vi "Get About Information.vi"(8 "error in (no error)":errorcluster) -> (0 "error out":errorcluster, 3 "About vCE text Out":string)   [LabVIEW 2013, in "FPGADMAChannelData.lvclass"]
uses:
  FPGADMAChannelData.lvclass
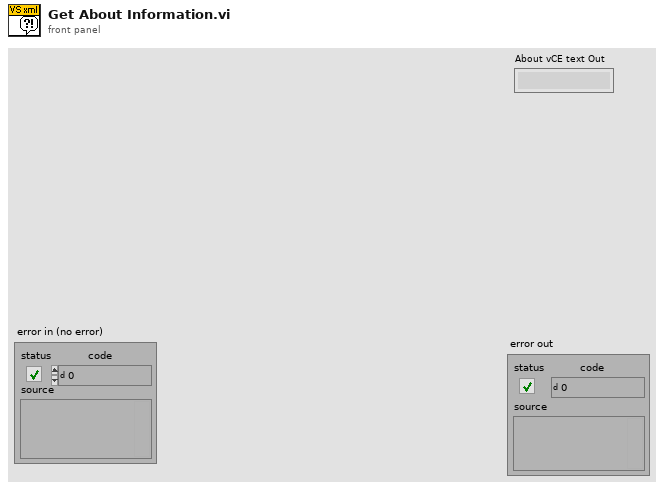
[diagram p1: front panel]
types:
  T1 = enum32{"invalid app kind", "Development System", "Run Time System", "Student Edition", "Embedded LabVIEW", "Evaluation", "Custom"}
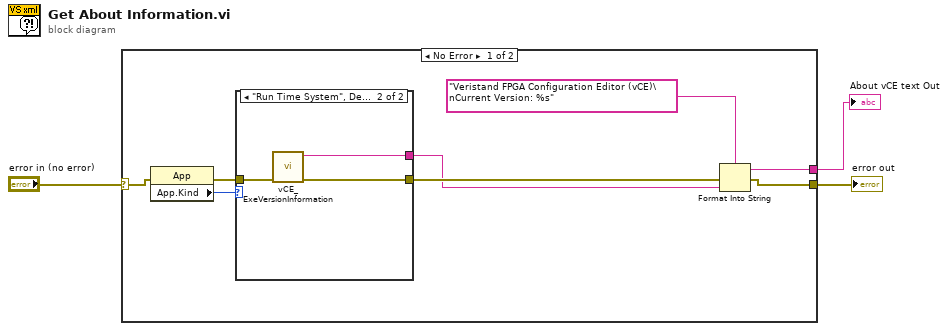
[diagram p0: block diagram]
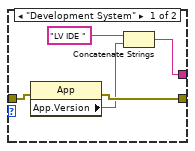
[diagram p2: hidden frame]
diagram:
  n1 = case shown="No Error" "error in (no error)" {
    selector: "error in (no error)" -> [w11 w20]
    tunnel: [w5 w20] -> w2
    tunnel: [w4 _] -> w1
    frame No Error {
      n2 = property class="App"(error in=w11) -> (error out=w9:errorcluster, "App.Kind"=w10:T1)  [unwired: 1 in, 1 out]
      n3 = case shown="\"Run Time System\", Default" w10 {
        tunnel: w9 -> [w16 w19]
        tunnel: [w15 w18] -> w8
        tunnel: [w12 w17] -> w7
        frame "Development System" {
          n4 = property class="App"(error in=w16) -> (error out=w15:errorcluster, "App.Version"=w13:string)  [unwired: 1 in, 1 out]
          n5 = Concatenate Strings("LV IDE " ("string"), w13) -> (w12:string)
        }
        frame "Run Time System", Default {
          n6 = call "vCE_ExeVersionInformation.vi"("error in (no error)"=w19) -> ("error out"=w18:errorcluster, "FileVersion"=w17:string)  [unwired: 9 in]
        }
      }
      n7 = Format Into String(format string="Veristand FPGA Configuration Editor (vCE)\nCurrent Version: %s", error in=w8, w7) -> (resulting string=w4:string, error out=w5:errorcluster)  [unwired: 1 in]
    }
    frame Error {
    }
  }
  "error out" <- w2
  "About vCE text Out" <- w1
